vi "Generate Datagridview value change event.vi"(8 "error in (no error)":errorcluster, 9 "DataGridView in":refnum<class "DataGridView.lvclass">, 10 "Datagridview ref":refnum<k24>, 11 "Event Registration Refnum":refnum<event-registration>) -> (0 "error out":errorcluster, 3 "Event Registration Refnum 2":refnum<event-registration>)   [LabVIEW 2013]
uses:
  System.Windows.Forms
  shared programs/LabVIEWdotNetDataGrid-master/source/DataGridView/DataGridView.lvclass
  shared programs/LabVIEWdotNetDataGrid-master/source/Events/Abstract EVENT/Abstract EVENT.lvclass
  shared programs/LabVIEWdotNetDataGrid-master/source/Events/CellValueChanged/CellValueChanged.lvclass
  shared programs/LabVIEWdotNetDataGrid-master/source/Events/CellValueChanged/CellValueChanged.lvclass/CellValueChanged.ctl
  shared programs/LabVIEWdotNetDataGrid-master/source/Events/CellValueChanged/Write row.vi
  shared programs/LabVIEWdotNetDataGrid-master/source/Events/CellValueChanged/Write column.vi
  shared programs/LabVIEWdotNetDataGrid-master/source/Events/CellValueChanged/Write cell value.vi
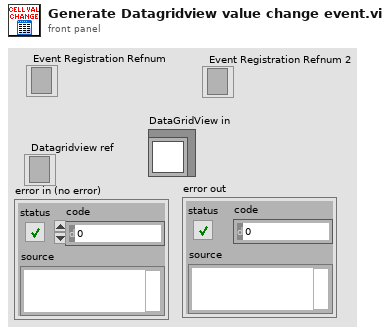
[diagram p1: front panel]
types:
  T1 = cluster{"CellClicked":refnum<user-event>, "CellValue Changed":refnum<user-event>, "KeyDown":refnum<user-event>, "DataError":refnum<user-event>, "UserAddedRow":refnum<user-event>, "UserDeletedRow":refnum<user-event>, "CellDirtyStateChanged":refnum<user-event>}
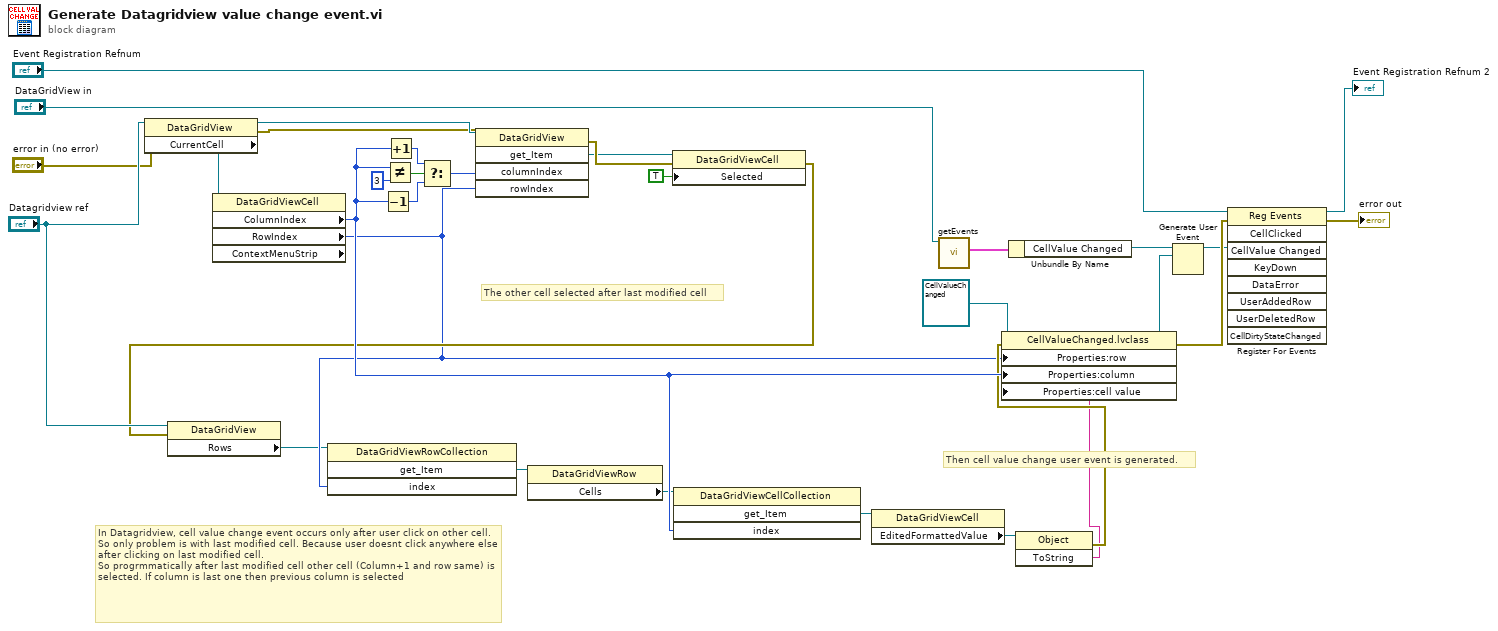
[diagram p0: block diagram]
diagram:
  # "Then cell value change user event is generated."
  # "In Datagridview, cell value change event occurs only after user click on other cell.\nSo only problem is with last modified cell. Because user doesnt click anywhere else after clicking on last modified cell.\nSo progrmmatically after last modified cell other cell (Column+1 and row same) is selected. If column is last one then previous column is selected"
  # "The other cell selected after last modified cell"
  n1 = property class="DataGridView"(reference="Datagridview ref", error in="error in (no error)") -> (reference out=w6:refnum<k24>, error out=w5:errorcluster, "CurrentCell"=w4:refnum<k24>)
  n2 = property class="DataGridViewCell" props=["ColumnIndex", "RowIndex", "ContextMenuStrip"](reference=w4) -> ("ColumnIndex"=w28:i32, "RowIndex"=w20:i32)  [unwired: 1 in, 3 out]
  n3 = Decrement(x=w28) -> (x-1=w29:i32)
  n4 = Not Equal?(x=w28, y=3) -> (x != y?=w26:bool)
  n5 = Increment(x=w28) -> (x+1=w27:i32)
  n6 = Select(t=w27, s=w26, f=w29) -> (s? t:f=w30:i32)
  n7 = invoke class="DataGridView" method="get_Item"(reference=w6, error in=w5, "columnIndex"=w30, "rowIndex"=w20) -> (error out=w14:errorcluster, "get_Item"=w12:refnum<k24>)  [unwired: 1 in, 3 out]
  n8 = property class="DataGridViewCell"(reference=w12, error in=w14, "Selected"=TRUE) -> (error out=w22:errorcluster)  [unwired: 1 out]
  n9 = property class="DataGridView"(reference="Datagridview ref", error in=w22) -> ("Rows"=w15:refnum<k24>)  [unwired: 2 out]
  n10 = invoke class="DataGridViewRowCollection" method="get_Item"(reference=w15, "index"=w20) -> ("get_Item"=w16:refnum<k24>)  [unwired: 2 in, 3 out]
  n11 = property class="DataGridViewRow"(reference=w16) -> ("Cells"=w17:refnum<k24>)  [unwired: 1 in, 2 out]
  n12 = invoke class="DataGridViewCellCollection" method="get_Item"(reference=w17, "index"=w28) -> ("get_Item"=w18:refnum<k24>)  [unwired: 2 in, 3 out]
  n13 = property class="DataGridViewCell"(reference=w18) -> ("EditedFormattedValue"=w19:refnum<k24>)  [unwired: 1 in, 2 out]
  n14 = call "getEvents.vi"("DataGridView in"="DataGridView in") -> ("userEvents"=w8:T1)  [unwired: 8 in, 2 out]
  n15 = Unbundle By Name(w8) -> ("CellValue Changed"=w9:refnum<user-event>)
  n16 = invoke class="Object" method="ToString"(reference=w19) -> (error out=w23:errorcluster, "ToString"=w21:string)  [unwired: 2 in, 1 out]
  n17 = property class="CellValueChanged.lvclass"(reference=refnum<class "CellValueChanged.lvclass"> refnum ("DataGrid.lvlib:CellValueChanged.lvclass"), error in=w23, "Properties:row"=w20, "Properties:column"=w28, "Properties:cell value"=w21) -> (reference out=w7:refnum<class "CellValueChanged.lvclass">, error out=w24:errorcluster)
  n18 = Generate User Event(user event=w9, event data cluster=w7) -> (user event out=w11:refnum<user-event>)  [unwired: 2 in, 1 out]
  n19 = register-events(reference="Event Registration Refnum", error in=w24, w11) -> (reference out=→"Event Registration Refnum 2":refnum<event-registration>, error out=→"error out":errorcluster)  [unwired: 6 in]
